vi "Simulated Device.vi"(8 "error in (no error)":errorcluster, 9 "Microcontroller":dbl, 10 "Channel":dbl, 11 "Simulated in":refnum<class "Simulated.lvclass">) -> (0 "error out":errorcluster, 1 "Response":string, 3 "Simulated out":refnum<class "Simulated.lvclass">)   [LabVIEW 2020, in "Simulated.lvclass"]
uses:
  Simulated.lvclass
  Abstract/Serial Device/Serial Device.lvclass
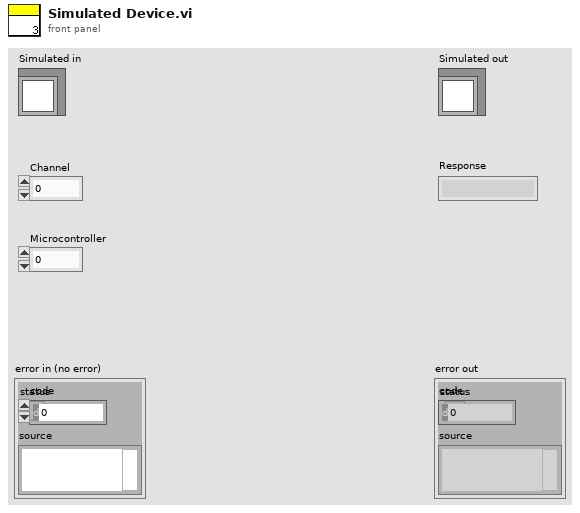
[diagram p1: front panel]
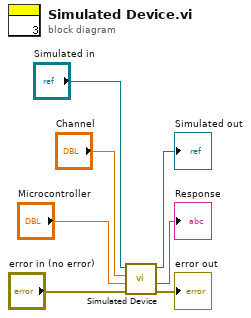
[diagram p0: block diagram]
diagram:
  n1 = call-parent "Simulated Device.vi"("error in (no error)"="error in (no error)", "Microcontroller"="Microcontroller", "Channel"="Channel", "Serial Device in"="Simulated in") -> ("error out"=→"error out":errorcluster, "Response"=→"Response":string, "Serial Device out"=→"Simulated out":refnum<class "Simulated.lvclass">)  [unwired: 5 in]
